vi "Read_binary_data.vi"() -> (1 "PWA Binary":i16[][](array[numeric]), 3 "PWA Frequency Hz":dbl format="%.2f", 5 "EOF?":bool, 6 "Block Header":string)   [LabVIEW 2017]
uses:
  Controls/Read I16 data cluster.ctl
  Globals/Meas_global.vi
  Globals/LDA_meas_global_1.vi
  Globals/LDA_meas_global_2.vi
panel:
  out "string":string
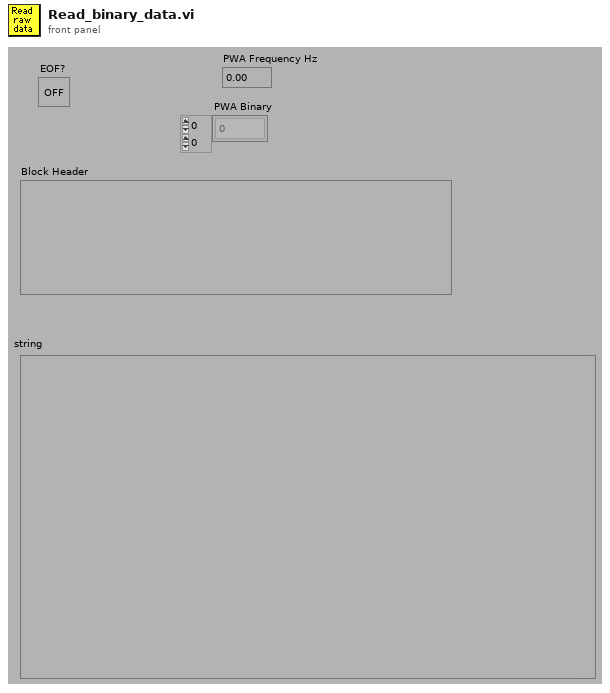
[diagram p1: front panel]
types:
  T1 = typedef "Analysis_info_cluster.ctl" = cluster{"Colour":u32, "Inst type":T2, "Inst name":string, "Symbol":string, "Code name":string, "Extra Info":string, "Inst Array":T3, "Extra Titles":string[], "Extra Values":string[], "U":dbl, "u^2":dbl, "u^3":dbl, "u^4":dbl, "Skew_u":dbl, "Kurt_u":dbl, "Sd Error in Mean":dbl, "% u'/U":dbl, "X":dbl, "Y":dbl, "Z":dbl, "Timescale integral Estimate":dbl, "Sd Error in Variance":dbl, "Calib File":path, "Calib Constants":dbl[], "Output Position":bool, "Full Stats":bool, "Av Sampling Rate":dbl, "Av No of Samples":dbl, "Total Meas Time (s)":dbl, "ADAM Ch Name":string, "Max value":dbl, "Min value":dbl, "Req Sample Rate Hz":dbl, "Sync Delay Time (s)":dbl, "Ch No":i16, "Device ID":string, "Use Latest Calib":bool, "Port":string}
  T2 = typedef "Inst_type.ctl" = enum16{"Propeller anemometer", "Raw voltage", "Pressure Transducer", "Pitot-static tube", "Preston tube", "Hot wire", "Cross wire 1", "Cross wire 2", "Generic Linear", "Generic Polynomial", "Generic BackPoly", "Fast FID", "Thermocouple", "Cold wire", "Pulsed Wire", "LDA Vel", "LDA Tran time", "LDA Arr time", "Microphone"}
  T3 = typedef "Instrument_Array.ctl" = enum16{"PWA", "LDA", "Analogue"}
  T4 = enum16{"read/write", "read-only", "write-only", "write-only (truncate)"}
  T5 = typedef "Read I16 data cluster.ctl" = cluster{"scale multiplier":dbl, "scale offset":dbl, "Length":i32, "Sampling rate (Hz)":dbl, "Sync Delay (s)":dbl}
  T6 = typedef "LDA_Setup.ctl" = cluster{"dimensions":enum16{"1D", "2D"}, "Sampling Rate Hz":dbl}
  T7 = typedef "BSA_Type.ctl" = enum16{"57N11", "BSA F60"}
  T8 = typedef "PWA_Data.ctl" = enum16{"No PWA Data", "One Ch PWA"}
  T9 = typedef "Time_Trace_Cluster.ctl" = cluster{"Weighting":dbl[], "Time (s)":dbl[], "Voltage":dbl[], "Eng Values":dbl[]}
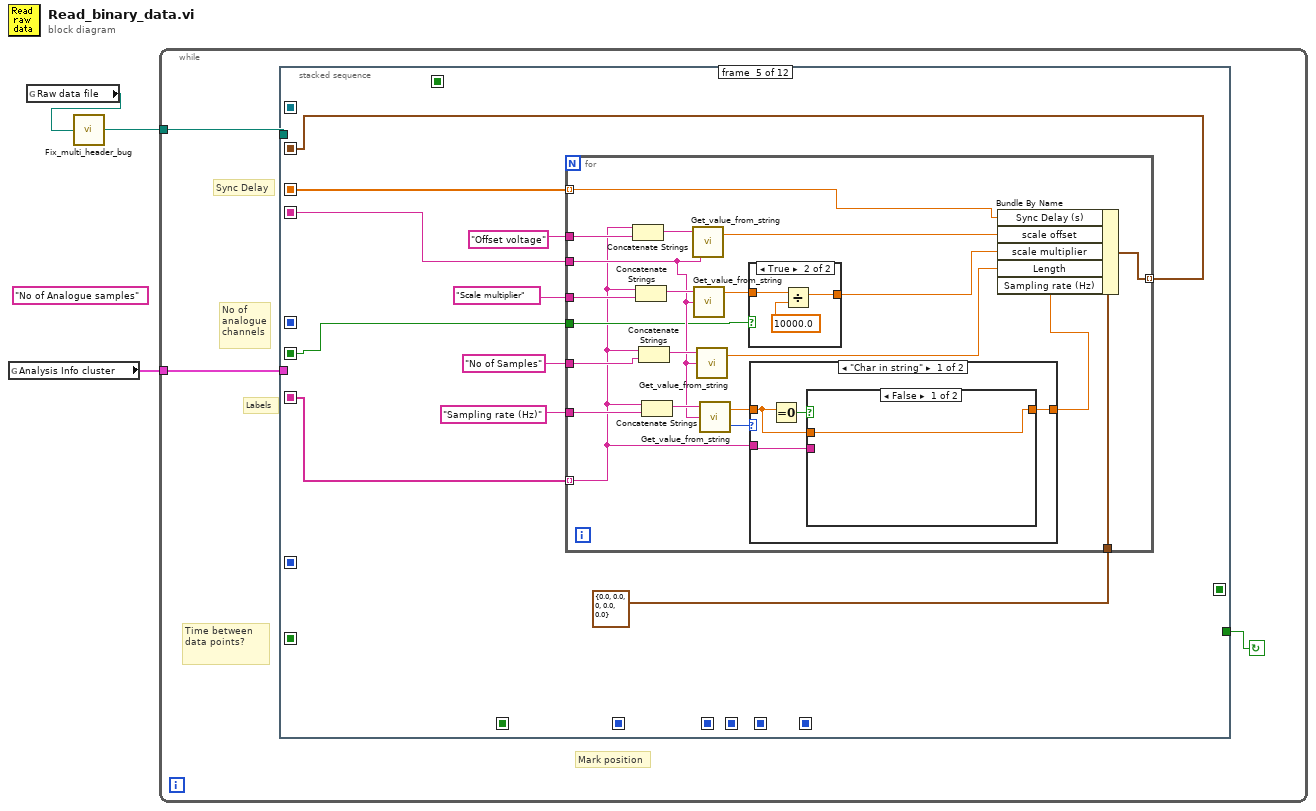
[diagram p0: block diagram]
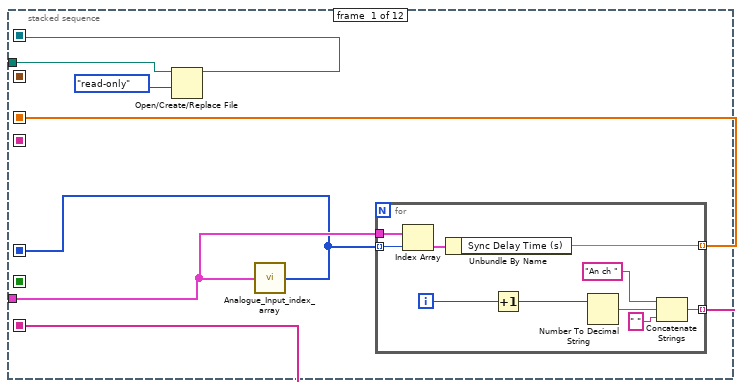
[diagram p2: hidden frame]
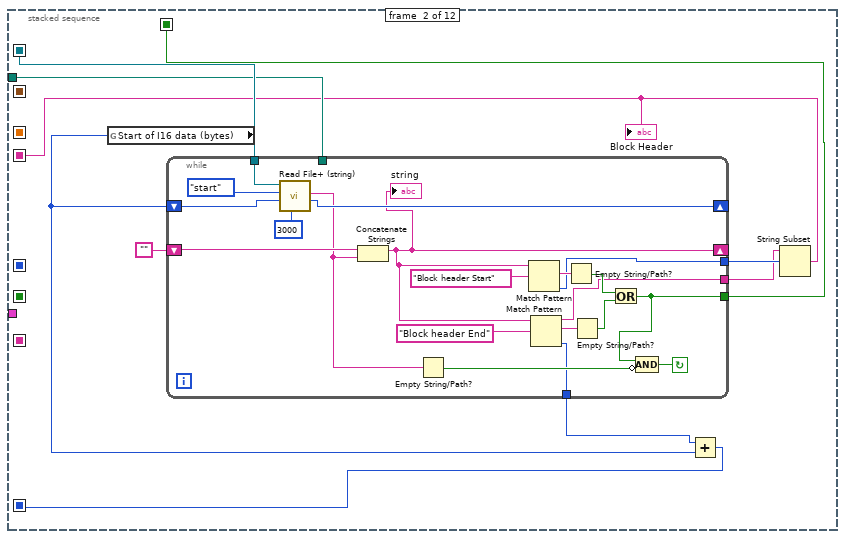
[diagram p3: hidden frame]
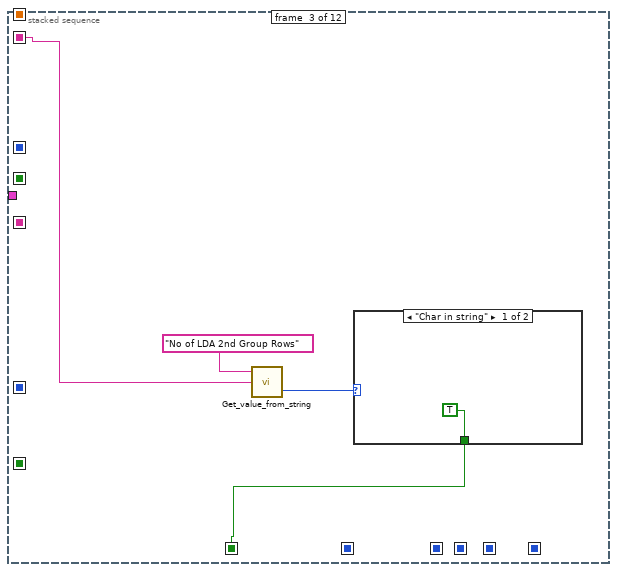
[diagram p4: hidden frame]
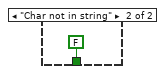
[diagram p5: hidden frame]
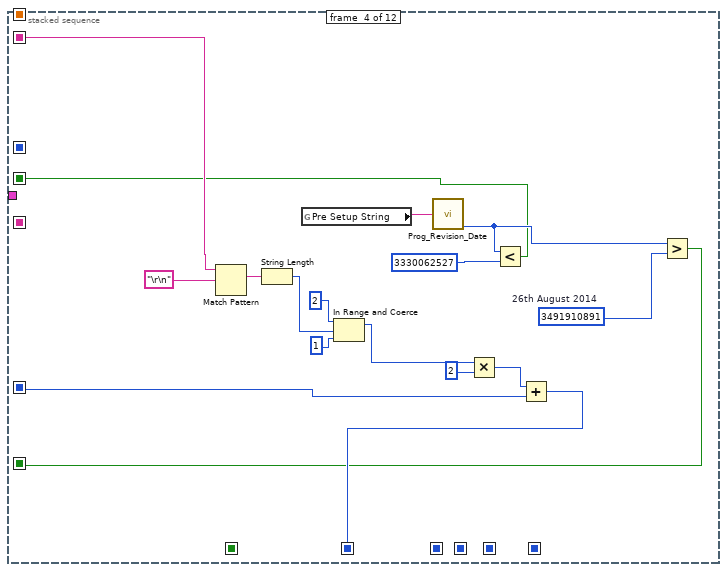
[diagram p6: hidden frame]
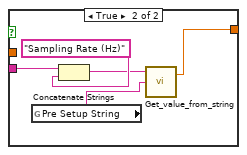
[diagram p7: hidden frame]
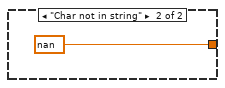
[diagram p8: hidden frame]
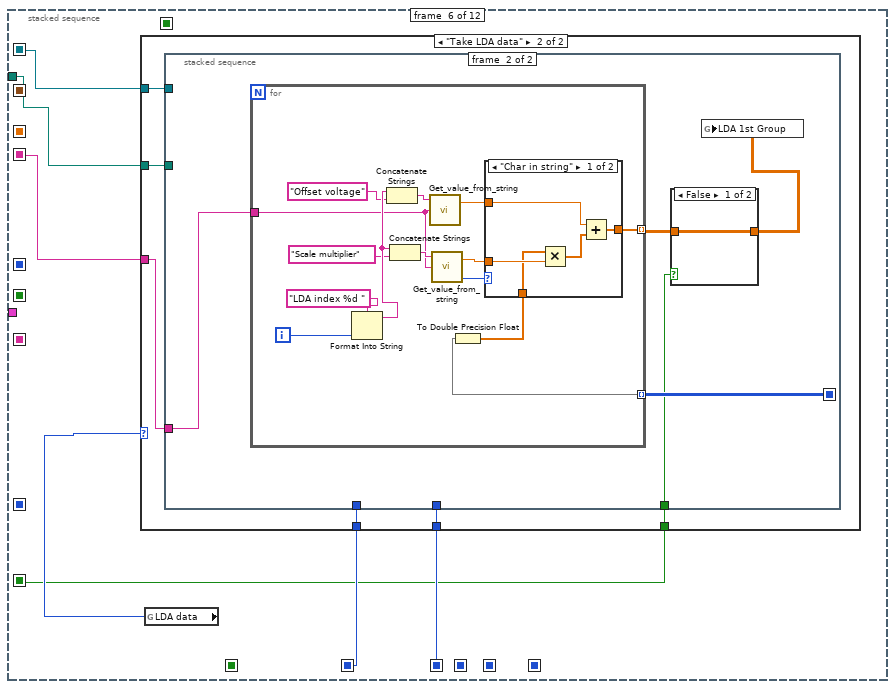
[diagram p10: hidden frame]
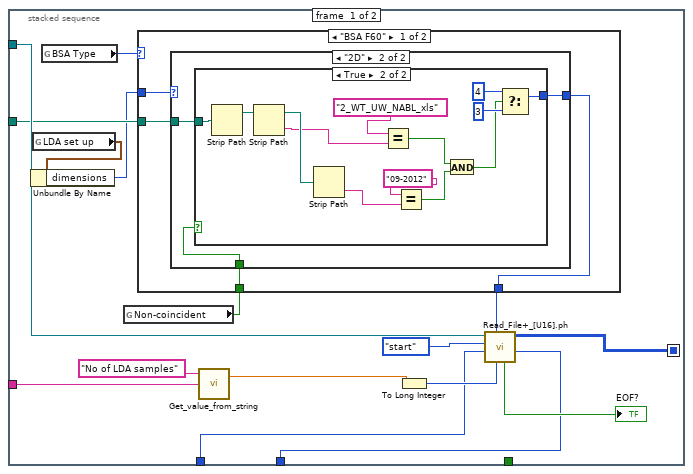
[diagram p12: hidden frame]
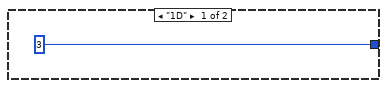
[diagram p13: hidden frame]
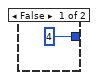
[diagram p14: hidden frame]
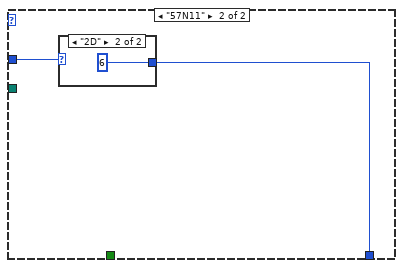
[diagram p15: hidden frame]
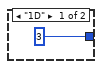
[diagram p16: hidden frame]
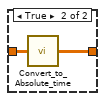
[diagram p17: hidden frame]
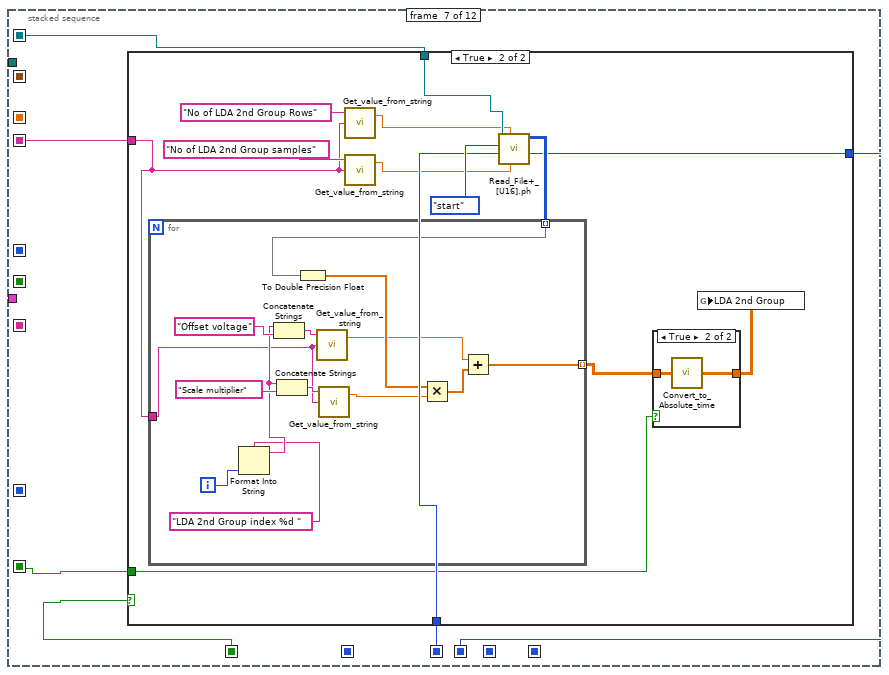
[diagram p19: hidden frame]
diagram:
  (unwired) "No of Analogue samples"
  n1 = global read "Meas_global.vi" "Analysis Info cluster"() -> (w1:T1[])
  n2 = global read "Meas_global.vi" "Raw data file"() -> (w3:path)
  n3 = call "Fix_multi_header_bug.vi"("Raw data File to Read"=w3) -> ("Raw data File to Read Out"=w2:path)
  n4 = while {
    tunnel: w2 -> [w6]
    tunnel: w1 -> [w4]
    stop <- w5 continue-if-true
    # "Sync Delay"
    # "Time between data points?"
    # "Mark position"
    # "Labels"
    # "No of\nanalogue\nchannels"
    n5 = stacked-sequence {
      seq-local: [w12 _ _ _ _ _ _ _ _ _ _ _] -> [_ w33 _ _ _ w126 w210 w249 w285 _ w316 w335]
      seq-local: [_ w24 _ _ _ _ _ _ _ _ _ _] -> [_ _ w56 w69 w82 w125 w211 w251 w280 w300 _ _]
      seq-local: [w7 _ _ _ _ _ _ _ _ _ _ _] -> [_ _ _ _ _ _ _ _ w279 _ _ _]
      seq-local: [w10 _ _ _ _ _ _ _ _ _ _ _] -> [_ _ _ _ w84 _ _ _ _ _ _ _]
      seq-local: [_ _ _ w74 _ _ _ _ _ _ _ _] -> [_ _ _ _ _ w128 _ _ _ _ _ _]
      seq-local: [_ _ _ _ _ w127 _ _ _ _ _ _] -> [_ _ _ _ _ _ w209 _ _ _ _ _]
      seq-local: [_ _ _ _ _ _ _ w250 _ _ _ _] -> [_ _ _ _ _ _ _ _ w283 _ _ _]
      seq-local: [_ w29 _ _ _ _ _ _ _ _ _ _] -> [_ _ _ _ _ _ _ _ _ _ _ w336]
      seq-local: [_ w28 _ _ _ _ _ _ _ _ _ _] -> [_ _ _ w75 _ _ _ _ _ _ _ _]
      seq-local: [_ _ _ _ _ _ _ _ _ w298 _ _] -> [_ _ _ _ _ _ _ _ _ _ w314 _]
      seq-local: [_ _ _ _ _ _ _ _ w282 _ _ _] -> [_ _ _ _ _ _ _ _ _ w297 w311 _]
      seq-local: [_ _ w54 _ _ _ _ _ _ _ _ _] -> [_ _ _ _ _ _ w212 _ _ _ _ _]
      seq-local: [_ _ _ _ _ _ w208 _ _ _ _ _] -> [_ _ _ _ _ _ _ w244 _ _ _ _]
      seq-local: [_ _ _ w61 _ _ _ _ _ _ _ _] -> [_ _ _ _ _ w123 w207 _ _ _ _ _]
      seq-local: [_ _ _ w60 _ _ _ _ _ _ _ _] -> [_ _ _ _ w81 _ _ _ _ _ _ _]
      seq-local: [_ _ _ _ w78 _ _ _ _ _ _ _] -> [_ _ _ _ _ _ _ _ w276 _ _ _]
      seq-local: [w9 _ _ _ _ _ _ _ _ _ _ _] -> [_ _ _ _ w77 _ _ _ _ _ _ _]
      tunnel: w6 -> [w11 w32 _ _ _ w124 _ _ _ _ _ w337]
      tunnel: [_ _ _ _ _ _ _ _ _ _ w312 _] -> w5
      tunnel: w4 -> [w8 _ _ _ _ _ _ _ _ _ _ _]
      frame #0 {
        n6 = Open/Create/Replace File(file path (use dialog)=w11, access (0:read/write)=T4."read-only" ("open mode (0)")) -> (refnum out=w12:refnum<file>)  [unwired: 1 in, 5 out]
        n7 = call "Analogue_Input_index_array.vi"("Analysis Info cluster"=w8) -> ("Array"=w7:i32[])
        n8 = for {
          tunnel: [w22] -> w10 mode=indexing
          tunnel: [w21] -> w9 mode=indexing
          tunnel: w8 -> [w16]
          tunnel: w7 -> [w15] mode=indexing
          i -> [w23]
          n9 = Index Array(array=w16, index=w15) -> (element=w14:T1)
          n10 = Unbundle By Name(w14) -> ("Sync Delay Time (s)"=w21:dbl)
          n11 = Increment(x=w23) -> (x+1=w18:i32)
          n12 = Number To Decimal String(number=w18) -> (decimal integer string=w20:string)  [unwired: 1 out]
          n13 = Concatenate Strings("An ch ", w20, " ") -> (w22:string)
        }
      }
      frame #1 {
        n14 = global read "Meas_global.vi" "Start of I16 data (bytes)"() -> (w30:i32)
        n15 = while {
          tunnel: [w38] -> w27
          tunnel: [w39] -> w29
          shift-left: "" -> [w42]
          shift-right: [w35] -> _
          tunnel: w32 -> [_]
          tunnel: w33 -> [w51]
          shift-left: w30 -> [w45]
          shift-right: [w50] -> _
          tunnel: [w37] -> w25
          tunnel: [w34] -> w26
          stop <- w46 continue-if-true
          n16 = call <vilib>:"Read File+ (string).vi"("count"=3000, "pos offset (bytes:0)"=w45, "pos mode (rel. to current:2)"=enum16{"start", "end", "current"}."start", "refnum"=w51) -> ("mark after read (bytes)"=w50:i32, "string"=w36:string)  [unwired: 1 in, 5 out]
          n17 = Concatenate Strings(w42, w36) -> (w35:string)
          "string" <- w35
          n18 = Empty String/Path?(string/path=w36) -> (empty?=w47:bool)
          n19 = Match Pattern(string=w35, regular expression="Block header Start") -> (match substring=w44:string, offset past match=w34:i32)  [unwired: 3 out]
          n20 = Match Pattern(string=w35, regular expression="Block header End") -> (before substring=w37:string, match substring=w52:string, offset past match=w38:i32)  [unwired: 2 out]
          n21 = Empty String/Path?(string/path=w44) -> (empty?=w41:bool)
          n22 = Empty String/Path?(string/path=w52) -> (empty?=w40:bool)
          n23 = Or(x=w41, y=w40) -> (x .or. y?=w39:bool)
          n24 = Compound Arithmetic op=AND(w39, invert w47) -> (w46:bool)
        }
        n25 = Add(x=w27, y=w30) -> (x+y=w28:i32)
        n26 = String Subset(string=w25, offset (0)=w26) -> (substring=w24:string)  [unwired: 1 out]
        "Block Header" <- w24
      }
      frame #2 {
        n27 = call "Get_value_from_string.vi"("Input string"=w56, "Variable name"="No of LDA 2nd Group Rows") -> ("Status"=w55:enum16{"Char in string", "Char not in string"})  [unwired: 1 in, 1 out]
        n28 = case shown="\"Char in string\"" w55 {
          tunnel: [TRUE FALSE] -> w54
          frame "Char in string" {
          }
          frame "Char not in string" {
          }
        }
      }
      frame #3 {
        w62 = u32 3491910891  # 26th August 2014
        n29 = Match Pattern(string=w69, regular expression="\r\n") -> (match substring=w68:string)  [unwired: 4 out]
        n30 = String Length(string=w68) -> (length=w67:i32)
        n31 = global read "Meas_global.vi" "Pre Setup String"() -> (w72:string)
        n32 = In Range and Coerce(upper limit=2, x=w67, lower limit=1) -> (coerced(x)=w66:i32)  [unwired: 1 out]
        n33 = call "Prog_Revision_Date.vi"("Input string"=w72) -> ("Revision time (s)"=w63:u32)  [unwired: 4 out]
        n34 = Multiply(x=w66, y=2) -> (x*y=w73:i32)
        n35 = Less?(x=w63, y=u32 3330062527 ("unsigned 32bit integer")) -> (x < y?=w60:bool)
        n36 = Add(x=w73, y=w75) -> (x+y=w74:i32)
        n37 = Greater?(x=w63, y=w62) -> (0:w61:bool)
      }
      frame #4 {
        n38 = for {
          tunnel: "Scale multiplier" -> [w107]
          tunnel: "Offset voltage" -> [w106]
          tunnel: w82 -> [w98]
          tunnel: w84 -> [w88] mode=indexing
          tunnel: T5 {"scale multiplier"=0.0, "scale offset"=0.0, "Length"=0, "Sampling rate (Hz)"=0.0, "Sync Delay (s)"=0.0} -> [w103]
          tunnel: "Sampling rate (Hz)" ("string") -> [w100]
          tunnel: "No of Samples" -> [w99]
          tunnel: w81 -> [w97]
          tunnel: [w90] -> w78 mode=indexing
          tunnel: w77 -> [w89] mode=indexing
          n39 = Concatenate Strings(w88, w106) -> (w105:string)
          n40 = Concatenate Strings(w88, w107) -> (w104:string)
          n41 = Concatenate Strings(w88, w99) -> (w102:string)
          n42 = Concatenate Strings(w88, w100) -> (w101:string)
          n43 = call "Get_value_from_string.vi"("Input string"=w98, "Variable name"=w105) -> ("Value"=w95:dbl)  [unwired: 1 in, 1 out]
          n44 = call "Get_value_from_string.vi"("Input string"=w98, "Variable name"=w104) -> ("Value"=w96:dbl)  [unwired: 1 in, 1 out]
          n45 = call "Get_value_from_string.vi"("Input string"=w98, "Variable name"=w102) -> ("Value"=w93:dbl)  [unwired: 1 in, 1 out]
          n46 = call "Get_value_from_string.vi"("Input string"=w98, "Variable name"=w101) -> ("Status"=w92:enum16{"Char in string", "Char not in string"}, "Value"=w91:dbl)  [unwired: 1 in]
          n47 = case shown="True" w97 {
            tunnel: w96 -> [w119 w122]
            tunnel: [w119 w120] -> w94
            frame False {
            }
            frame True {
              n48 = Divide(x=w122, y=10000.0) -> (x/y=w120:dbl)
            }
          }
          n49 = case shown="\"Char in string\"" w92 {
            tunnel: [w109 nan ("Value")] -> w87
            tunnel: w91 -> [w108 _]
            tunnel: w88 -> [w111 _]
            frame "Char in string" {
              n50 = Equal To 0?(x=w108) -> (x = 0?=w110:bool)
              n51 = case shown="False" w110 {
                tunnel: w111 -> [_ w117]
                tunnel: [w112 w113] -> w109
                tunnel: w108 -> [w112 _]
                frame False {
                }
                frame True {
                  n52 = global read "Meas_global.vi" "Pre Setup String"() -> (w115:string)
                  n53 = Concatenate Strings(w117, "Sampling Rate (Hz)" ("string")) -> (w114:string)
                  n54 = call "Get_value_from_string.vi"("Input string"=w115, "Variable name"=w114) -> ("Value"=w113:dbl)  [unwired: 1 in, 1 out]
                }
              }
            }
            frame "Char not in string" {
            }
          }
          n55 = Bundle By Name(cluster=w103, "Sync Delay (s)"=w89, "scale offset"=w95, "scale multiplier"=w94, "Length"=w93, "Sampling rate (Hz)"=w87) -> (w90:T5)
        }
      }
      frame #5 {
        n56 = global read "Meas_global.vi" "LDA data"() -> (w129:enum16{"No LDA data", "Take LDA data"})
        n57 = case shown="\"Take LDA data\"" w129 {
          tunnel: w125 -> [_ w134]
          tunnel: w128 -> [w130 w135]
          tunnel: [w130 w133] -> w127
          tunnel: w126 -> [_ w136]
          tunnel: w124 -> [_ w132]
          tunnel: w123 -> [_ w131]
          frame "No LDA data" {
          }
          frame "Take LDA data" {
            n58 = stacked-sequence {
              seq-local: [w139 _] -> [_ w182]
              tunnel: w136 -> [w152 _]
              tunnel: w135 -> [w144 _]
              tunnel: w134 -> [w143 w183]
              tunnel: [w141 _] -> w133
              tunnel: w132 -> [w140 _]
              tunnel: w131 -> [_ w179]
              frame #0 {
                n59 = global read "Meas_global.vi" "LDA set up"() -> (w138:T6)
                n60 = Unbundle By Name(w138) -> ("dimensions"=w137:enum16{"1D", "2D"})
                n61 = global read "LDA_meas_global_1.vi" "BSA Type"() -> (w146:T7)
                n62 = global read "LDA_meas_global_1.vi" "Non-coincident"() -> (w142:bool)
                n63 = case shown="\"BSA F60\"" w146 {
                  tunnel: w137 -> [w156 w176]
                  tunnel: [w154 w175] -> w145
                  tunnel: w142 -> [w155 _]
                  tunnel: w140 -> [w153 _]
                  frame "BSA F60" {
                    n64 = case shown="\"2D\"" w156 {
                      tunnel: [3 w160] -> w154
                      tunnel: w155 -> [_ w159]
                      tunnel: w153 -> [_ w158]
                      frame "1D" {
                      }
                      frame "2D" {
                        n65 = case shown="True" w159 {
                          tunnel: [4 w172] -> w160
                          tunnel: w158 -> [_ w171]
                          frame False {
                          }
                          frame True {
                            n66 = Strip Path(path=w171) -> (stripped path=w169:path)  [unwired: 1 out]
                            n67 = Strip Path(path=w169) -> (stripped path=w170:path, name=w166:string)
                            n68 = Strip Path(path=w170) -> (name=w165:string)  [unwired: 1 out]
                            n69 = Equal?(x="2_WT_UW_NABL_xls", y=w166) -> (x = y?=w163:bool)
                            n70 = Equal?(x="09-2012", y=w165) -> (x = y?=w164:bool)
                            n71 = And(x=w163, y=w164) -> (x .and. y?=w162:bool)
                            n72 = Select(t=4, s=w162, f=3) -> (s? t:f=w172:i32)
                          }
                        }
                      }
                    }
                  }
                  frame "57N11" {
                    n73 = case shown="\"2D\"" w176 {
                      tunnel: [3 6] -> w175
                      frame "1D" {
                      }
                      frame "2D" {
                      }
                    }
                  }
                }
                n74 = call "Get_value_from_string.vi"("Input string"=w143, "Variable name"="No of LDA samples") -> ("Value"=w150:dbl)  [unwired: 1 in, 1 out]
                n75 = To Long Integer(number=w150) -> (32bit integer=w148:i32)
                n76 = call "Read_File+_[U16].ph.vi"("2D number of columns/1D count"=w148, "2D number of rows"=w145, "pos offset (bytes:0)"=w144, "pos mode (rel. to current:2)"=enum16{"start", "end", "current"}."start", "refnum"=w152) -> ("mark after read (bytes)"=w141:i32, "2D data"=w139:u16[][], "EOF?"=→"EOF?":bool)  [unwired: 1 in, 3 out]
              }
              frame #1 {
                n77 = for {
                  tunnel: w183 -> [w192]
                  tunnel: w182 -> [w190] mode=indexing
                  tunnel: [w188] -> w181 mode=indexing
                  i -> [w191]
                  n78 = Format Into String(format string="LDA index %d ", w191) -> (resulting string=w197:string)  [unwired: 2 in, 1 out]
                  n79 = Concatenate Strings(w197, "Offset voltage") -> (w194:string)
                  n80 = Concatenate Strings(w197, "Scale multiplier") -> (w193:string)
                  n81 = call "Get_value_from_string.vi"("Input string"=w192, "Variable name"=w194) -> ("Value"=w198:dbl)  [unwired: 1 in, 1 out]
                  n82 = call "Get_value_from_string.vi"("Input string"=w192, "Variable name"=w193) -> ("Status"=w187:enum16{"Char in string", "Char not in string"}, "Value"=w200:dbl)  [unwired: 1 in]
                  n83 = To Double Precision Float(number=w190) -> (double precision float=w189:dbl[])
                  n84 = case shown="\"Char in string\"" w187 {
                    tunnel: w200 -> [w205 _]
                    tunnel: w198 -> [w204 _]
                    tunnel: w189 -> [w202 w206]
                    tunnel: [w201 w206] -> w188
                    frame "Char in string" {
                      n85 = Multiply(x=w202, y=w205) -> (x*y=w203:dbl[])
                      n86 = Add(x=w204, y=w203) -> (x+y=w201:dbl[])
                    }
                    frame "Char not in string" {
                    }
                  }
                }
                n87 = case shown="False" w179 {
                  tunnel: w181 -> [w184 w186]
                  tunnel: [w184 w185] -> w180
                  frame False {
                  }
                  frame True {
                    n88 = call "Convert_to_Absolute_time.vi"("LDA Group in"=w186) -> ("LDA Group out"=w185:dbl[][])
                  }
                }
                n89 = global write "LDA_meas_global_2.vi" "LDA 1st Group"(w180) -> ()
              }
            }
          }
        }
      }
      frame #6 {
        n90 = case shown="True" w212 {
          tunnel: w211 -> [_ w221]
          tunnel: w210 -> [_ w223]
          tunnel: w209 -> [w213 w222]
          tunnel: [w213 w219] -> w208
          tunnel: w207 -> [_ w216]
          frame False {
          }
          frame True {
            n91 = call "Get_value_from_string.vi"("Input string"=w221, "Variable name"="No of LDA 2nd Group Rows") -> ("Value"=w218:dbl)  [unwired: 1 in, 1 out]
            n92 = call "Get_value_from_string.vi"("Input string"=w221, "Variable name"="No of LDA 2nd Group samples") -> ("Value"=w217:dbl)  [unwired: 1 in, 1 out]
            n93 = call "Read_File+_[U16].ph.vi"("2D number of columns/1D count"=w217, "2D number of rows"=w218, "pos offset (bytes:0)"=w222, "pos mode (rel. to current:2)"=enum16{"start", "end", "current"}."start", "refnum"=w223) -> ("mark after read (bytes)"=w219:i32, "2D data"=w220:u16[][])  [unwired: 1 in, 4 out]
            n94 = for {
              tunnel: w221 -> [w238]
              tunnel: w220 -> [w231] mode=indexing
              tunnel: [w230] -> w215 mode=indexing
              i -> [w234]
              n95 = Format Into String(format string="LDA 2nd Group index %d ", w234) -> (resulting string=w239:string)  [unwired: 2 in, 1 out]
              n96 = Concatenate Strings(w239, "Offset voltage") -> (w242:string)
              n97 = Concatenate Strings(w239, "Scale multiplier") -> (w243:string)
              n98 = To Double Precision Float(number=w231) -> (double precision float=w237:dbl[])
              n99 = call "Get_value_from_string.vi"("Input string"=w238, "Variable name"=w242) -> ("Value"=w235:dbl)  [unwired: 1 in, 1 out]
              n100 = call "Get_value_from_string.vi"("Input string"=w238, "Variable name"=w243) -> ("Value"=w233:dbl)  [unwired: 1 in, 1 out]
              n101 = Multiply(x=w237, y=w233) -> (x*y=w236:dbl[])
              n102 = Add(x=w235, y=w236) -> (x+y=w230:dbl[])
            }
            n103 = case shown="True" w216 {
              tunnel: w215 -> [w227 w229]
              tunnel: [w227 w228] -> w214
              frame False {
              }
              frame True {
                n104 = call "Convert_to_Absolute_time.vi"("LDA Group in"=w229) -> ("LDA Group out"=w228:dbl[][])
              }
            }
            n105 = global write "LDA_meas_global_2.vi" "LDA 2nd Group"(w214) -> ()
          }
        }
      }
      frame #7 {
        n106 = global read "Meas_global.vi" "PWA Data"() -> (w247:T8)
        n107 = case shown="\"No PWA Data\"" w247 {
          tunnel: [0 1] -> w246
          frame "No PWA Data" {
          }
          frame "One Ch PWA" {
          }
        }
        n108 = Not Equal To 0?(x=w246) -> (x != 0?=w248:bool)
        n109 = case shown="True" w248 {
          tunnel: w251 -> [_ w256]
          tunnel: w244 -> [w255 w264]
          tunnel: [w255 w266] -> w250
          tunnel: w249 -> [_ w270]
          tunnel: w246 -> [_ w269]
          tunnel: [i16[][] [] ("2D array") w265] -> w245
          frame False {
          }
          frame True {
            w260 = FALSE  # Show Dialog?
            n110 = call "Get_Characters_from_string.vi"("Input string"=w256, "Variable name"="No of PWA samples") -> ("Value"=w263:string)  [unwired: 1 in, 1 out]
            n111 = Decimal String To Number(string=w263) -> (number=w262:i32)  [unwired: 3 out]
            n112 = call <vilib>:"Read File+ [I16].vi"("2D number of columns/1D count"=w262, "2D number of rows"=w269, "pos offset (bytes:0)"=w264, "pos mode (rel. to current:2)"=enum16{"start", "end", "current"}."start", "refnum"=w270) -> ("mark after read (bytes)"=w266:i32, "2D data"=w265:i16[][], "EOF?"=w267:bool)  [unwired: 1 in, 3 out]
            n113 = local write "EOF?"(w267) -> ()
            n114 = call "Get_value_from_string.vi"("Show Dialog?"=w260, "Input string"=w256, "Variable name"="ADC Frequency Hz") -> ("Status"=w257:enum16{"Char in string", "Char not in string"}, "Value"=w259:dbl)
            n115 = case shown="\"Char not in string\"" w257 {
              tunnel: w259 -> [w272 _]
              tunnel: [w272 w273] -> w258
              tunnel: w256 -> [_ w274]
              frame "Char in string" {
              }
              frame "Char not in string" {
                n116 = call "Get_value_from_string.vi"("Input string"=w274, "Variable name"="Actual sampling rate") -> ("Value"=w273:dbl)  [unwired: 1 in, 1 out]
              }
            }
            "PWA Frequency Hz" <- w258
          }
        }
        "PWA Binary" <- w245
      }
      frame #8 {
        n117 = global read "Meas_global.vi" "Time Trace"() -> (w278:T9[])
        n118 = Array Size(array=w279) -> (size(s)=w281:i32)
        n119 = Not Equal To 0?(x=w281) -> (x != 0?=w284:bool)
        n120 = case shown="True" w284 {
          tunnel: w280 -> [_ w288]
          tunnel: w283 -> [w287 w294]
          tunnel: [w287 w295] -> w282
          tunnel: w285 -> [_ w296]
          tunnel: w279 -> [_ w293]
          tunnel: w278 -> [w286 w292]
          tunnel: [w286 w290] -> w277
          tunnel: w276 -> [_ w289]
          frame False {
          }
          frame True {
            n121 = call "Read I16 analogue Data.vi"("Block Header"=w288, "Channel info"=w289, "Time Trace In"=w292, "Anaologue Index"=w293, "pos offset (bytes:0)"=w294, "refnum"=w296) -> ("Time Trace out"=w290:T9[], "EOF?"=w291:bool, "mark after read (bytes)"=w295:i32)  [unwired: 3 in]
            n122 = local write "EOF?"(w291) -> ()
          }
        }
        n123 = global write "Meas_global.vi" "Time Trace"(w277) -> ()
      }
      frame #9 {
        n124 = global read "Meas_global.vi" "Blocks to Skip"() -> (w299:i32[])
        n125 = Array Size(array=w299) -> (size(s)=w302:i32)
        n126 = Equal To 0?(x=w302) -> (x = 0?=w301:bool)
        n127 = case shown="False" w301 {
          tunnel: w300 -> [w308 _]
          tunnel: w299 -> [w305 _]
          tunnel: [w303 FALSE] -> w298
          frame False {
            n128 = call "Get_value_from_string.vi"("Input string"=w308, "Variable name"="Block No") -> ("Value"=w307:dbl)  [unwired: 1 in, 1 out]
            n129 = To Long Integer(number=w307) -> (32bit integer=w306:i32)
            n130 = Search 1D Array(1D array=w305, element=w306) -> (index of element=w304:i32)  [unwired: 1 out]
            n131 = Greater Or Equal To 0?(x=w304) -> (x >= 0?=w303:bool)
          }
          frame True {
          }
        }
        n132 = global write "Meas_global.vi" "Start of I16 data (bytes)"(w297) -> ()
      }
      frame #10 {
        n133 = local read "EOF?"() -> (w315:bool)
        n134 = case shown="False" w315 {
          tunnel: w311 -> [w319 _]
          tunnel: w316 -> [w318 _]
          tunnel: [w317 w333] -> w313
          tunnel: w315 -> [_ w333]
          frame False {
            n135 = while {
              tunnel: [w323] -> w317
              tunnel: w318 -> [w330]
              shift-left: w319 -> [w325]
              shift-right: [w326] -> _
              stop <- w321 continue-if-true
              n136 = call <vilib>:"Read File+ (string).vi"("count"=3000, "pos offset (bytes:0)"=w325, "pos mode (rel. to current:2)"=enum16{"start", "end", "current"}."start", "refnum"=w330) -> ("error out"=w324:errorcluster, "mark after read (bytes)"=w326:i32, "string"=w327:string, "EOF?"=w320:bool)  [unwired: 1 in, 3 out]
              n137 = Unbundle By Name(w324) -> ("status"=w322:bool)
              n138 = Match Pattern(string=w327, regular expression="Block header") -> (match substring=w331:string)  [unwired: 4 out]
              n139 = Empty String/Path?(string/path=w331) -> (empty?=w323:bool)
              n140 = Compound Arithmetic op=AND(w323, invert w322, invert w320) -> (w321:bool)
            }
          }
          frame True {
          }
        }
        n141 = local write "EOF?"(w313) -> ()
        n142 = Compound Arithmetic op=AND(w314, invert w313) -> (w312:bool)
      }
      frame #11 {
        n143 = Close File(refnum=w335) -> (error out=w334:errorcluster)  [unwired: 1 in, 1 out]
        n144 = case shown="True" w336 {
          tunnel: w337 -> [w340 _]
          tunnel: w334 -> [w338 _]
          frame False {
            n145 = call "Add_filename_to_err_message.vi"("error in (no error)"=w338, "Path"=w340) -> ("error out"=w341:errorcluster)
            n146 = call "EnFlo_Error_Handler.vi"("error in (no error)"=w341, "Dialog Box (T)"=TRUE) -> ()  [unwired: 1 in, 3 out]
          }
          frame True {
            w345 = FALSE  # Dialog Box
            n147 = Bundle By Name(cluster=errorcluster {"status"=FALSE, "code"=0, "source"=""} ("error in (no error)"), "status"=TRUE ("Bundle Element"), "source"="The block header was not found in the file" ("Bundle Element")) -> (w346:errorcluster)
            n148 = call "EnFlo_Error_Handler.vi"("error in (no error)"=w346, "Error Type"="Raw Data File Error", "Dialog Box (T)"=w345) -> ()  [unwired: 3 out]
          }
        }
      }
    }
  }
